vi "CSMKVMap-Write.vi"(5 "name":string, 6 "Error in":errorcluster caption="Error in (no error)", 9 "value":variant) -> (0 "Error out":errorcluster)   [LabVIEW 2017, in "Communicable State Machine.lvlib"]
uses:
  ChangeFlag/ChangeFlag-Write.vi
  Utility/Random Change Flag.vi
  ChangeFlag/ChangeFlagDB.vi
  CSMKVMapDVR.vi
  Communicable State Machine.lvlib
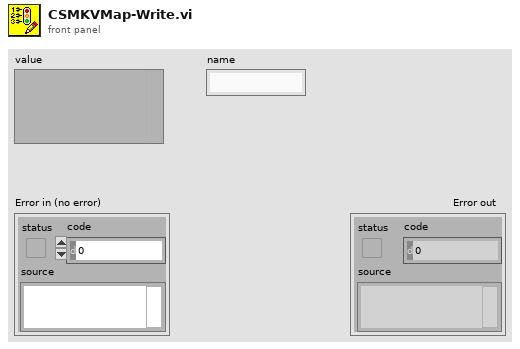
[diagram p1: front panel]
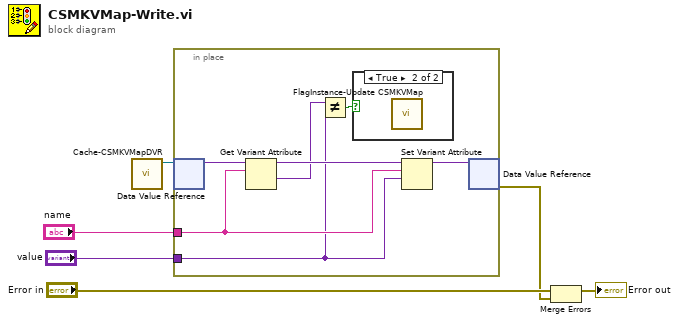
[diagram p0: block diagram]
diagram:
  n1 = call "Cache-CSMKVMapDVR.vi"() -> ("KVMapDVR"=w1:refnum<data-value>)  [unwired: 11 in]
  n2 = in-place {
    in-place-border: "name" -> [w9]
    in-place-border: "value" -> [w8]
    n3 = in-place-dvr #1(w1) -> (w13:variant)  [unwired: 1 out]
    n4 = Get Variant Attribute(Variant=w13, name=w9) -> (duplicate Variant=w11:variant, value=w10:variant)  [unwired: 2 in, 2 out]
    n5 = Not Equal?(x=w10, y=w8) -> (x != y?=w7:bool)
    n6 = case shown="True" w7 {
      frame False {
      }
      frame True {
        n7 = call "FlagInstance-Update CSMKVMap.vi"() -> ()  [unwired: 10 in, 2 out]
      }
    }
    n8 = Set Variant Attribute(Variant=w11, name=w9, value=w8) -> (Variant out=w12:variant)  [unwired: 1 in, 2 out]
    n9 = in-place-dvr #1(w12) -> (w3:errorcluster)  [unwired: 1 out]
  }
  n10 = Merge Errors("Error in", w3) -> (→"Error out":errorcluster)
